vi "Initialize_Serial_Device_2.0.vi"(8 "error in (no error)":errorcluster, 10 "Enum":enum16{"Arduino Uno", "Pump", "Arduino Mega"}(ring), 11 "Data":T1 {"SystemVersion" items=["Standard", "XL"]; "Tap1" items=["Session Data", "Extended Setup", "Buffer", "Camera", "Dispenser", "Stats", "Connections"]; "I don't think is in use"."Light intensity" scale=0.0..100.0; "Camera settings"."Crop settings"."Cam2"."Rectangle 2"."Rotation" format="%.2f"; "Camera settings"."Crop settings"."Cam2"."Rectangle 2"."Left" scale=0.0..1024.0; "Camera settings"."Crop settings"."Cam2"."Rectangle 2"."Right" scale=0.0..1024.0; "Camera settings"."Crop settings"."Cam1"."Rectangle 1"."Rotation" format="%.2f"; "Camera settings"."Crop settings"."Cam1"."Rectangle 1"."Left" scale=0.0..1024.0; "Camera settings"."Crop settings"."Cam1"."Rectangle 1"."Right" scale=0.0..1024.0; "Camera settings"."Lens/camera settings"."Framerate" min=1; "Camera settings"."Lens/camera settings"."Max Framerate" min=1; "Camera settings"."Detection settings"."Sample size threshold" min=1; "Pump"."Flush Size" min=0 max=6000 step=100; "Ques"."Overload threshold" min=1; "Ques"."Image Save Queue Size" min=1; "Ques"."Image Process Queue Size" min=1}) -> (0 "error out":errorcluster, 2 "Connection":bool, 3 "Data 2":T1={"Camera 1"={"Camera1"="", "Cam 1"=FALSE, "CAM1 Model"=enum."a2A5328-15ucBAS", "Cam1 ID"=0}, "Camera 2"={"Camera2"="", "Cam 2"=FALSE, "CAM2 Model"=enum."a2A5328-15ucBAS", "Cam2 ID"=0}, "Image"={"Camera1_Img"=refnum, "Camera2_Img"=refnum, "Img1_Orig_Disp"=refnum, "Img2_Orig_Disp"=refnum, "Img1_Orig_RGB"=refnum, "Img2_Orig_RGB"=refnum, "Blue_Plane_Extract"=refnum, "Subtracted_Plane"=refnum, "Img1_Binary"=refnum, "Img2_Binary"=refnum, "Crop_Mask"=refnum, "Img1_Save"=refnum, "Img2_Save"=refnum, "Img1_Cali_Full"=refnum, "Img2_Cali_Full"=refnum, "Img1_Cali_Detect"=refnum, "Img2_Cali_Detect"=refnum}, "Ques"={"Cam 1 queue"=refnum, "Cam 2 queue"=refnum, "Cam 1 - save queue"=refnum, "Cam 2 - save queue"=refnum, "Image Process Queue Size"=500, "Image Save Queue Size"=500, "Overload threshold"=500, "Max large object threshold"=0}, "Arduino SRS"={"Pinch-valve"="", "Actuator"=FALSE, "Open(T)/Close(F)"=FALSE, "Arduino Uno"=""}, "Pump"={"Port"="", "Connection"=FALSE, "Flush Size"=0, "Command"="", "Pump Size"=enum."Large", "Pump"="", "Ready"=FALSE}, "Camera settings"={"Detection settings"={"Sample size threshold"=500, "Detection Region %"=30.0, "Timeout Sample"=200}, "Lens/camera settings"={"Aperture"=enum."Item 0", "Legacy Cam Attributes"=FALSE, "Max Framerate"=100, "Exposure Time"=1000.0, "Framerate"=15}, "Crop settings"={"Cam1"={"Rectangle 1"={"Left"=0, "Top"=0, "Right"=0, "Bottom"=0, "Rotation"=0.0}, "Camera Orientation 1"="", "Pixel to mm 1"=0.0}, "Cam2"={"Rectangle 2"={"Left"=0, "Top"=0, "Right"=0, "Bottom"=0, "Rotation"=0.0}, "Camera Orientation 2"="", "Pixel to mm 2"=0.0}}}, "Arduino ISS"={"Mega F3"="", "Phase3"=FALSE, "Barcode"="", "Sorting sys."=FALSE, "Initial size"=0.0, "Size Interval"=0.0, "Mun. of containers"=0.0, "Container nr."=0.0, "Arduino Mega"=""}, "Img_Capt"=FALSE, "Empty_Refill"=FALSE, "I don't think is in use"={"Light intensity"=100}, "Extended setup"={"Location"="Station", "Latitude"="Station", "Longitude"="Station", "Determiner"="Station", "Sex"="Station", "Station"="", "Collection date"=""}, "Main interface"={"Sample Name"="Test Sample", "Operator"="JFR", "Species Name"="", "Other Notes"=""}, "Tap1"=0, "SystemVersion"=0, "System Serial"="", "Exit"=FALSE, "Kuvette Full"=FALSE, "Core JKI"={"Current VI Reference"=refnum, "Close Panel on Exit?"=FALSE}, "Calibration"={"Calibration 1"=path "C:/Users/au540322/Desktop/IHS_Project/images/Debris/Debris_0/Debris_0_2019_06_01-23-32-49-686.PNG", "Calibration 2"=path "C:/Users/au540322/Desktop/IHS_Project/images/Debris/Debris_0/Debris_0_2019_06_01-23-32-49-686.PNG", "Detect 1"=path "C:/Users/au540322/Desktop/IHS_Project/images/Debris/Debris_0/Debris_0_2019_06_01-23-32-49-686.PNG", "Detect 2"=path "C:/Users/au540322/Desktop/IHS_Project/images/Debris/Debris_0/Debris_0_2019_06_01-23-32-49-686.PNG"}, "Auto Flush"=FALSE} {"SystemVersion" items=["Standard", "XL"]; "Tap1" items=["Session Data", "Extended Setup", "Buffer", "Camera", "Dispenser", "Stats", "Connections"]; "I don't think is in use"."Light intensity" scale=0.0..100.0; "Camera settings"."Crop settings"."Cam2"."Rectangle 2"."Rotation" format="%.2f"; "Camera settings"."Crop settings"."Cam2"."Rectangle 2"."Left" scale=0.0..1024.0; "Camera settings"."Crop settings"."Cam2"."Rectangle 2"."Right" scale=0.0..1024.0; "Camera settings"."Crop settings"."Cam1"."Rectangle 1"."Rotation" format="%.2f"; "Camera settings"."Crop settings"."Cam1"."Rectangle 1"."Left" scale=0.0..1024.0; "Camera settings"."Crop settings"."Cam1"."Rectangle 1"."Right" scale=0.0..1024.0; "Camera settings"."Lens/camera settings"."Framerate" min=1; "Camera settings"."Lens/camera settings"."Max Framerate" min=1; "Camera settings"."Detection settings"."Sample size threshold" min=1; "Pump"."Flush Size" min=0 max=6000 step=100; "Ques"."Overload threshold" min=1; "Ques"."Image Save Queue Size" min=1; "Ques"."Image Process Queue Size" min=1})   [LabVIEW 2024]
uses:
  controls/Data_JKI.ctl
  <vilib>/userDefined/High Color/IMAQdx.ctl
  <vilib>/vision/Image Controls.llb/IMAQ Image.ctl
  <vilib>/Instr/_visa.llb/VISA Find Search Mode.ctl
  b9f502e1-47a6-4cec-8472-59ce789a2094.vi
  24558789-6baa-4d89-876d-522026fff3d8.vi
  9ba94584-cf90-4084-937e-f244570da27e.vi
  19e22268-0b19-48d3-ab11-a72bc7dea378.vi
  <vilib>/regexp/Match Regular Expression.xnode
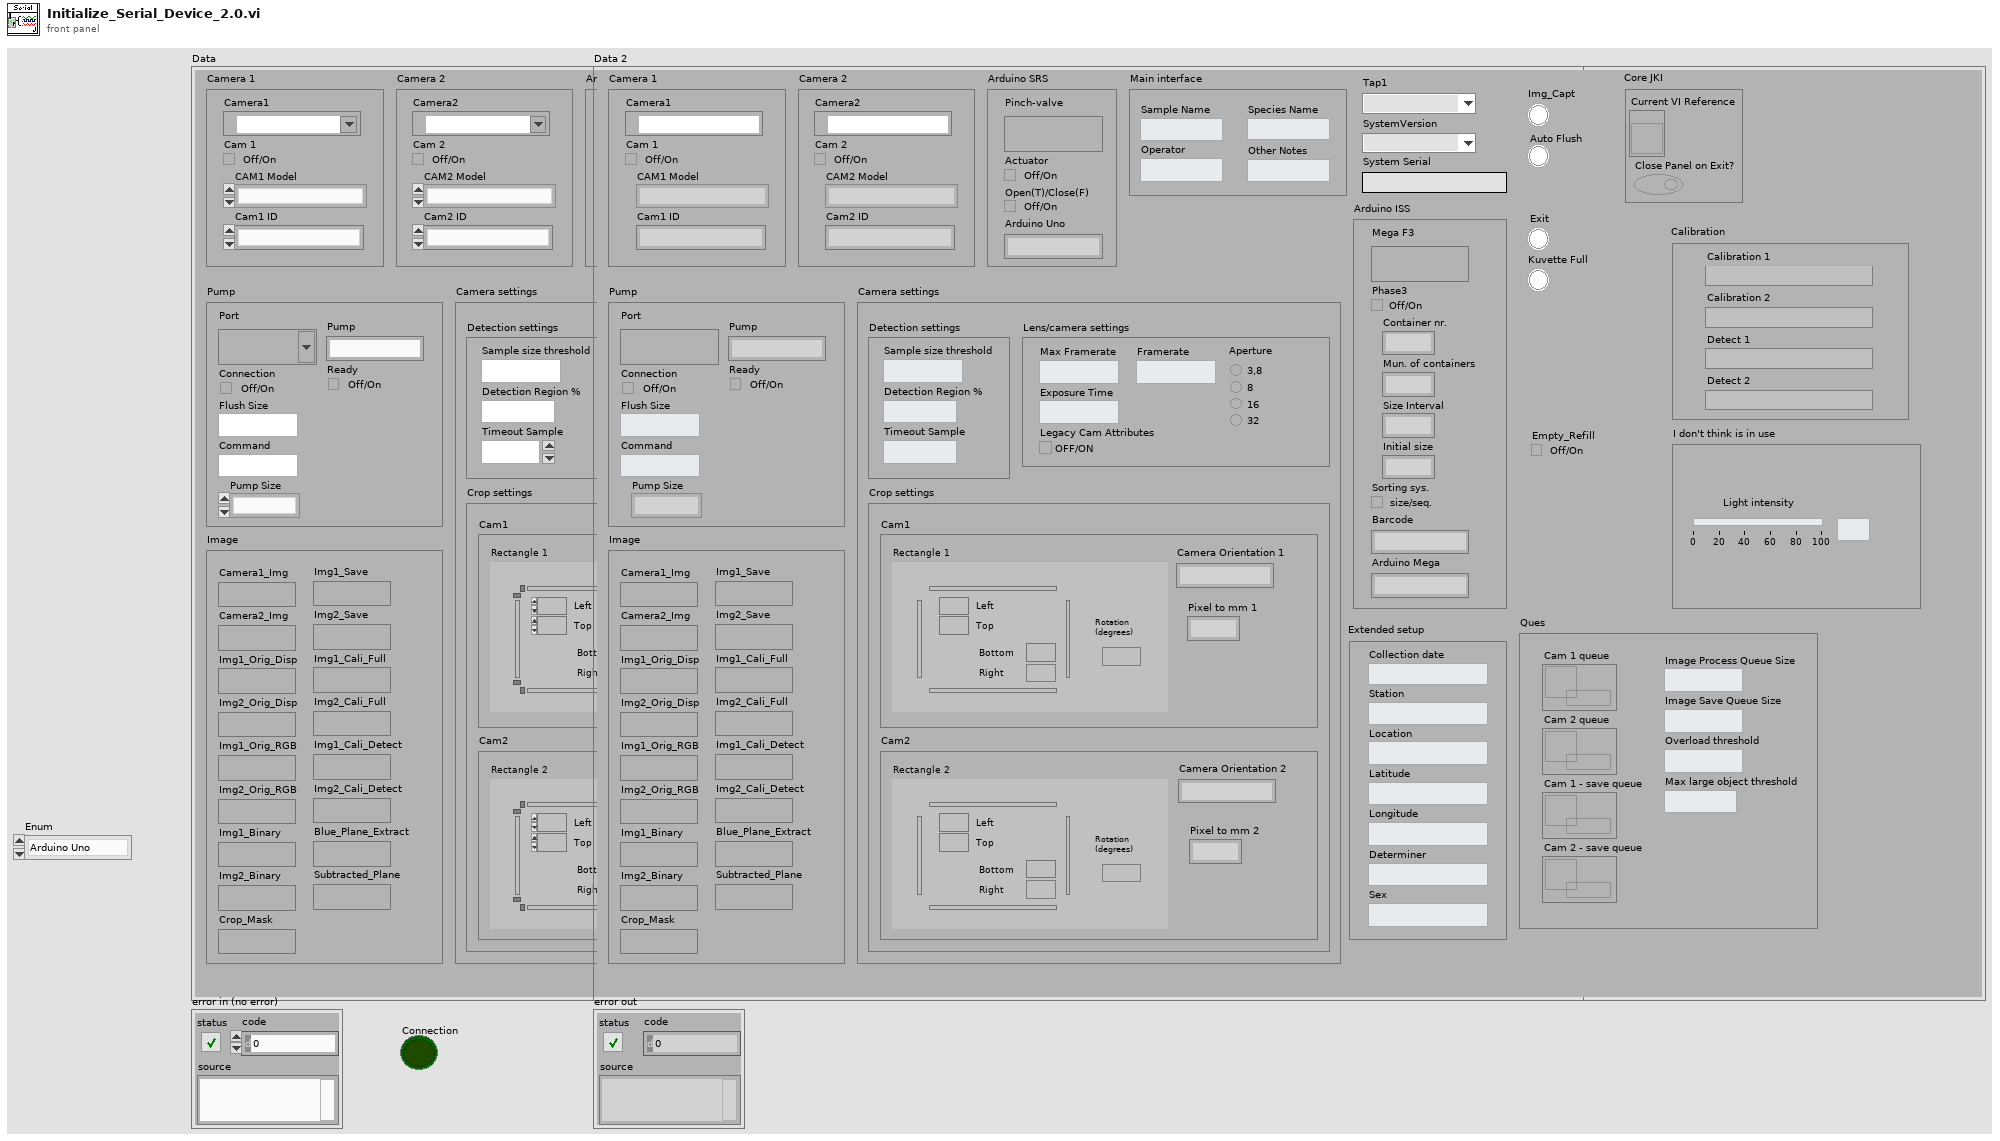
[diagram p1: front panel]
types:
  T1 = typedef "Data_JKI.ctl" = cluster{"Camera 1":cluster{"Camera1":T2, "Cam 1":bool, "CAM1 Model":enum16{"a2A5328-15ucBAS", "acA1920-155uc"}, "Cam1 ID":i32}, "Camera 2":cluster{"Camera2":T2, "Cam 2":bool, "CAM2 Model":enum16{"a2A5328-15ucBAS", "acA1920-155uc"}, "Cam2 ID":i32}, "Image":cluster{"Camera1_Img":T3, "Camera2_Img":T3, "Img1_Orig_Disp":T3, "Img2_Orig_Disp":T3, "Img1_Orig_RGB":T3, "Img2_Orig_RGB":T3, "Blue_Plane_Extract":T3, "Subtracted_Plane":T3, "Img1_Binary":T3, "Img2_Binary":T3, "Crop_Mask":T3, "Img1_Save":T3, "Img2_Save":T3, "Img1_Cali_Full":T3, "Img2_Cali_Full":T3, "Img1_Cali_Detect":T3, "Img2_Cali_Detect":T3}, "Ques":cluster{"Cam 1 queue":refnum<queue>, "Cam 2 queue":refnum<queue>, "Cam 1 - save queue":refnum<queue>, "Cam 2 - save queue":refnum<queue>, "Image Process Queue Size":i32, "Image Save Queue Size":i32, "Overload threshold":i32, "Max large object threshold":i32}, "Arduino SRS":cluster{"Pinch-valve":refnum<visa-resource-name>, "Actuator":bool, "Open(T)/Close(F)":bool, "Arduino Uno":string}, "Pump":cluster{"Port":refnum<visa-resource-name>, "Connection":bool, "Flush Size":i32, "Command":string, "Pump Size":enum16{"None", "Small", "Large"}, "Pump":string, "Ready":bool}, "Camera settings":cluster{"Detection settings":cluster{"Sample size threshold":i32, "Detection Region %":dbl, "Timeout Sample":i32}, "Lens/camera settings":cluster{"Aperture":enum32{"Item 0", "Item 1", "Item 2", "Item 3"}, "Legacy Cam Attributes":bool, "Max Framerate":i32, "Exposure Time":dbl, "Framerate":i32}, "Crop settings":cluster{"Cam1":cluster{"Rectangle 1":T4, "Camera Orientation 1":string, "Pixel to mm 1":dbl}, "Cam2":cluster{"Rectangle 2":T4, "Camera Orientation 2":string, "Pixel to mm 2":dbl}}}, "Arduino ISS":cluster{"Mega F3":refnum<visa-resource-name>, "Phase3":bool, "Barcode":string, "Sorting sys.":bool, "Initial size":dbl, "Size Interval":dbl, "Mun. of containers":dbl, "Container nr.":dbl, "Arduino Mega":string}, "Img_Capt":bool, "Empty_Refill":bool, "I don't think is in use":cluster{"Light intensity":i32}, "Extended setup":cluster{"Location":string, "Latitude":string, "Longitude":string, "Determiner":string, "Sex":string, "Station":string, "Collection date":string}, "Main interface":cluster{"Sample Name":string, "Operator":string, "Species Name":string, "Other Notes":string}, "Tap1":u16, "SystemVersion":u16, "System Serial":string, "Exit":bool, "Kuvette Full":bool, "Core JKI":cluster{"Current VI Reference":refnum<vi>, "Close Panel on Exit?":bool}, "Calibration":cluster{"Calibration 1":path, "Calibration 2":path, "Detect 1":path, "Detect 2":path}, "Auto Flush":bool}
  T2 = typedef "IMAQdx.ctl" = refnum<k21>
  T3 = typedef "IMAQ Image.ctl" = refnum<image>
  T4 = typedef "IMAQ Rectangle" = cluster{"Left":i32, "Top":i32, "Right":i32, "Bottom":i32, "Rotation":dbl}
  T5 = typedef "VISA Find Search Mode.ctl" = u32
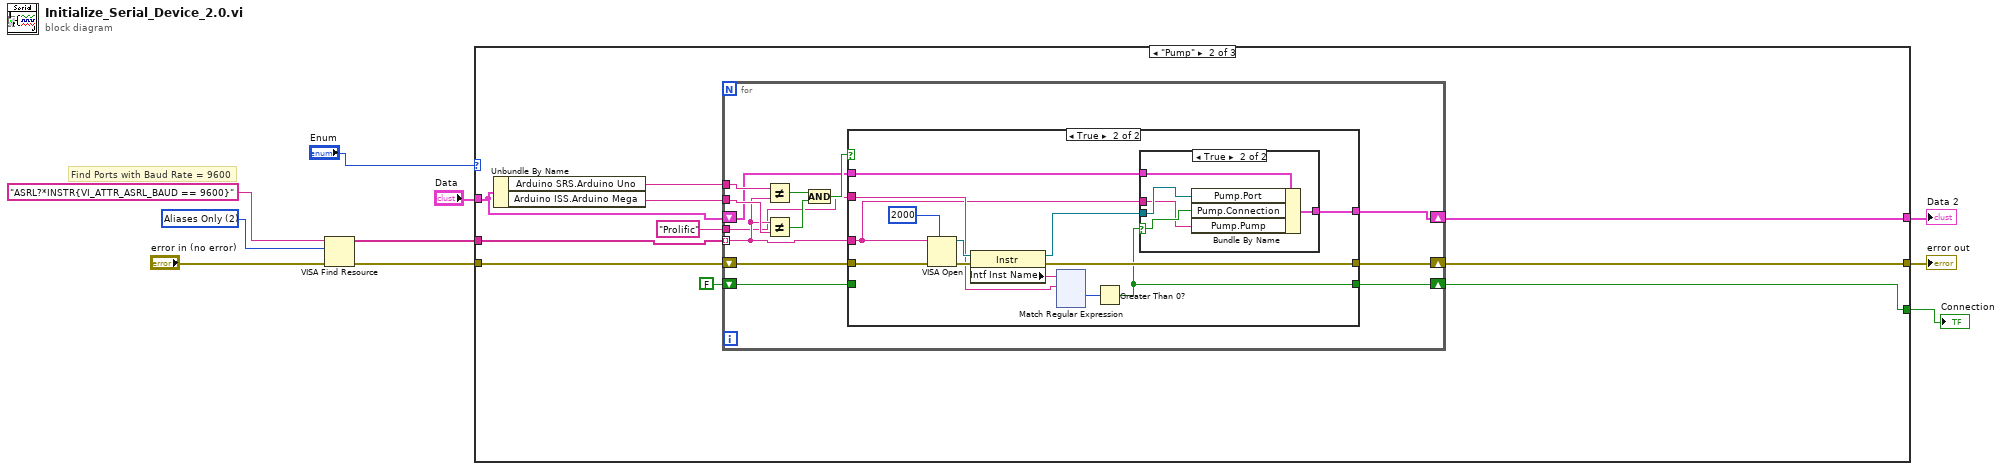
[diagram p0: block diagram]
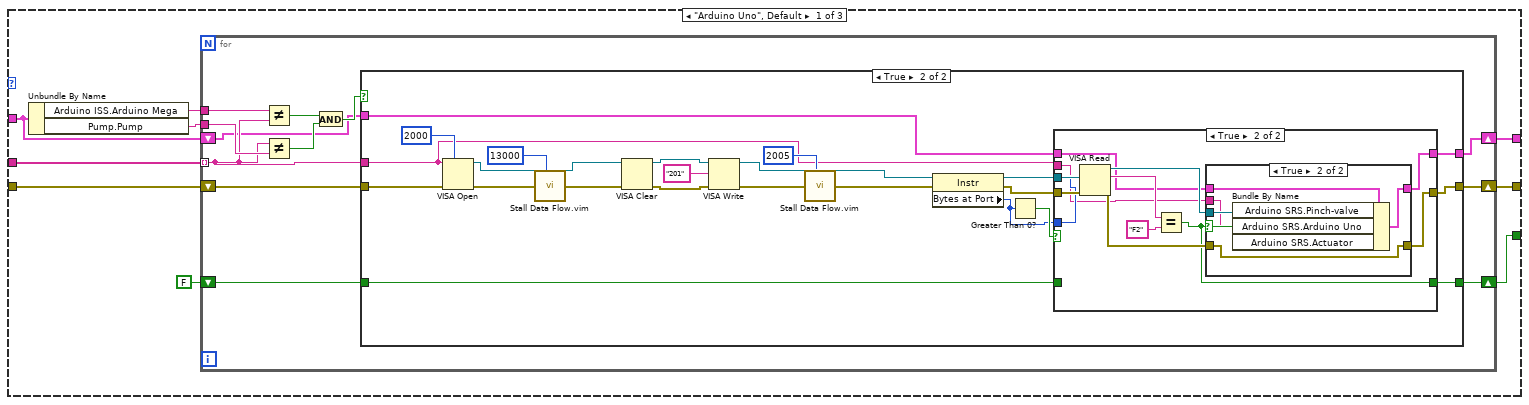
[diagram p2: hidden frame]
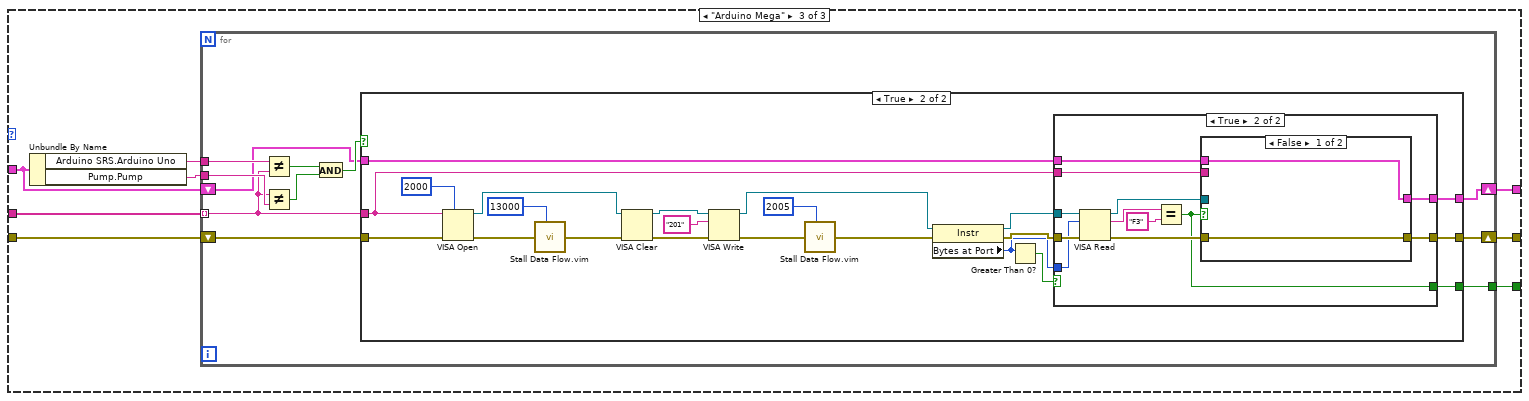
[diagram p8: hidden frame]
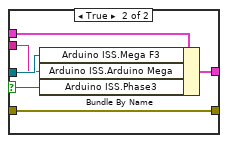
[diagram p11: hidden frame]
diagram:
  w10 = T5 2 items=["Canonical Names Only"=0, "Aliases Only"=2, "Include Matching Aliases"=3, "Include All Aliases"=4] ("Search Mode")
  # "Find Ports with Baud Rate = 9600"
  n1 = VISA Find Resource(8:"error in (no error)", 10:w10, 11:"ASRL?*INSTR{VI_ATTR_ASRL_BAUD == 9600}" ("expression (\"?*\")")) -> (0:w7:errorcluster, 3:w8:string[])  [unwired: 1 out]
  n2 = case shown="\"Pump\"" "Enum" {
    tunnel: w8 -> [w17 w90 w245]
    tunnel: w7 -> [w15 w86 w244]
    tunnel: "Data" -> [w16 w85 w246]
    tunnel: [w14 w84 w247] -> w5
    tunnel: [w13 w83 w248] -> w4
    tunnel: [w12 w82 w243] -> w1
    frame "Arduino Uno", Default {
      n3 = Unbundle By Name(w16) -> ("Arduino ISS.Arduino Mega"=w19:string, "Pump.Pump"=w18:string)
      n4 = for {
        tunnel: w17 -> [w29] mode=indexing
        tunnel: w19 -> [w31]
        tunnel: w18 -> [w30]
        shift-right: [w25] -> w14
        shift-left: w16 -> [w24]
        shift-right: [w22] -> w13
        shift-left: w15 -> [w23]
        shift-right: [w21] -> w12
        shift-left: FALSE -> [w20]
        n5 = Not Equal?(x=w31, y=w29) -> (x != y?=w28:bool)
        n6 = Not Equal?(x=w29, y=w30) -> (x != y?=w27:bool)
        n7 = And(x=w28, y=w27) -> (x .and. y?=w26:bool)
        n8 = case shown="True" w26 {
          tunnel: w29 -> [_ w38]
          tunnel: w24 -> [w34 w39]
          tunnel: [w34 w37] -> w25
          tunnel: w23 -> [w33 w43]
          tunnel: [w33 w40] -> w22
          tunnel: [w32 w36] -> w21
          tunnel: w20 -> [w32 w35]
          frame False {
          }
          frame True {
            n9 = VISA Open(timeout (0)=u32 2000 ("VISA Open timeout (0)"), error in (no error)=w43, VISA resource name=w38) -> (VISA resource name=w42:refnum<visa-resource-name>, error out=w41:errorcluster)  [unwired: 2 in]
            n10 = call "Stall Data Flow.vim"("value in"=w41, "milliseconds to wait"=u32 13000) -> ("value out"=w46:errorcluster)  [unwired: 1 out]
            n11 = VISA Clear(VISA resource name=w42, error in (no error)=w46) -> (VISA resource name out=w56:refnum<visa-resource-name>, error out=w57:errorcluster)
            n12 = VISA Write(VISA resource name=w56, write buffer="201", error in (no error)=w57) -> (VISA resource name out=w54:refnum<visa-resource-name>, error out=w49:errorcluster)  [unwired: 1 out]
            n13 = call "Stall Data Flow.vim"("value in"=w49, "milliseconds to wait"=u32 2005) -> ("value out"=w48:errorcluster)  [unwired: 1 out]
            n14 = property class="Instr"(reference=w54, error in=w48) -> (reference out=w52:refnum<visa-resource-name>, error out=w51:errorcluster, "Bytes at Port"=w50:u32)
            n15 = Greater Than 0?(x=w50) -> (x > 0?=w53:bool)
            n16 = case shown="True" w53 {
              tunnel: w52 -> [_ w72]
              tunnel: w51 -> [w59 w71]
              tunnel: w50 -> [_ w70]
              tunnel: [w59 w66] -> w40
              tunnel: w39 -> [w60 w64]
              tunnel: w38 -> [_ w63]
              tunnel: [w60 w62] -> w37
              tunnel: [w58 w61] -> w36
              tunnel: w35 -> [w58 _]
              frame False {
              }
              frame True {
                n17 = VISA Read(VISA resource name=w72, byte count=w70, error in (no error)=w71) -> (VISA resource name out=w65:refnum<visa-resource-name>, read buffer=w69:string, error out=w67:errorcluster)  [unwired: 1 out]
                n18 = Equal?(x=w69, y="F2") -> (x = y?=w61:bool)
                n19 = case shown="True" w61 {
                  selector: w61 -> [_ w77]
                  tunnel: [w73 w80] -> w66
                  tunnel: w67 -> [w73 w80]
                  tunnel: w65 -> [_ w78]
                  tunnel: w64 -> [w74 w79]
                  tunnel: w63 -> [_ w76]
                  tunnel: [w74 w75] -> w62
                  frame False {
                  }
                  frame True {
                    n20 = Bundle By Name(cluster=w79, "Arduino SRS.Pinch-valve"=w78, "Arduino SRS.Arduino Uno"=w76, "Arduino SRS.Actuator"=w77) -> (w75:T1)
                  }
                }
              }
            }
          }
        }
      }
    }
    frame "Pump" {
      n21 = Unbundle By Name(w85) -> ("Arduino SRS.Arduino Uno"=w89:string, "Arduino ISS.Arduino Mega"=w87:string)
      n22 = for {
        tunnel: w90 -> [w101] mode=indexing
        tunnel: w89 -> [w103]
        tunnel: "Prolific" -> [w97]
        tunnel: w87 -> [w102]
        shift-right: [w96] -> w84
        shift-left: w85 -> [w95]
        shift-right: [w93] -> w83
        shift-left: w86 -> [w94]
        shift-right: [w92] -> w82
        shift-left: FALSE -> [w91]
        n23 = Not Equal?(x=w103, y=w101) -> (x != y?=w100:bool)
        n24 = Not Equal?(x=w101, y=w102) -> (x != y?=w99:bool)
        n25 = And(x=w100, y=w99) -> (x .and. y?=w98:bool)
        n26 = case shown="True" w98 {
          tunnel: w101 -> [_ w108]
          tunnel: w97 -> [_ w114]
          tunnel: w95 -> [w106 w113]
          tunnel: [w106 w111] -> w96
          tunnel: w94 -> [w105 w110]
          tunnel: [w105 w109] -> w93
          tunnel: [w104 w107] -> w92
          tunnel: w91 -> [w104 _]
          frame False {
          }
          frame True {
            n27 = VISA Open(timeout (0)=u32 2000 ("VISA Open timeout (0)"), error in (no error)=w110, VISA resource name=w108) -> (VISA resource name=w119:refnum<visa-resource-name>, error out=w116:errorcluster)  [unwired: 2 in]
            n28 = property class="Instr"(reference=w119, error in=w116) -> (reference out=w112:refnum<visa-resource-name>, error out=w109:errorcluster, "Intf Inst Name"=w115:string)
            n29 = xnode "Match Regular Expression"("input string"=w115, "regular expression"=w114) -> ("offset past match"=w118:i32)  [unwired: 4 in, 4 out]
            n30 = Greater Than 0?(x=w118) -> (x > 0?=w107:bool)
            n31 = case shown="True" w107 {
              selector: w107 -> [_ w124]
              tunnel: w113 -> [w120 w125]
              tunnel: w112 -> [_ w123]
              tunnel: [w120 w122] -> w111
              tunnel: w108 -> [_ w121]
              frame False {
              }
              frame True {
                n32 = Bundle By Name(cluster=w125, "Pump.Port"=w123, "Pump.Connection"=w124, "Pump.Pump"=w121) -> (w122:T1)
              }
            }
          }
        }
      }
    }
    frame "Arduino Mega" {
      n33 = Unbundle By Name(w246) -> ("Arduino SRS.Arduino Uno"=w250:string, "Pump.Pump"=w249:string)
      n34 = for {
        tunnel: w245 -> [w259] mode=indexing
        tunnel: w250 -> [w261]
        tunnel: w249 -> [w260]
        shift-right: [w255] -> w247
        shift-left: w246 -> [w254]
        shift-right: [w252] -> w248
        shift-left: w244 -> [w253]
        tunnel: [w251] -> w243
        n35 = Not Equal?(x=w261, y=w259) -> (x != y?=w258:bool)
        n36 = Not Equal?(x=w259, y=w260) -> (x != y?=w257:bool)
        n37 = And(x=w258, y=w257) -> (x .and. y?=w256:bool)
        n38 = case shown="True" w256 {
          selector: w256 -> [w262 _]
          tunnel: w259 -> [_ w267]
          tunnel: w254 -> [w264 w268]
          tunnel: [w264 w266] -> w255
          tunnel: w253 -> [w263 w272]
          tunnel: [w263 w269] -> w252
          tunnel: [w262 w265] -> w251
          frame False {
          }
          frame True {
            n39 = VISA Open(timeout (0)=u32 2000 ("VISA Open timeout (0)"), error in (no error)=w272, VISA resource name=w267) -> (VISA resource name=w271:refnum<visa-resource-name>, error out=w270:errorcluster)  [unwired: 2 in]
            n40 = call "Stall Data Flow.vim"("value in"=w270, "milliseconds to wait"=u32 13000) -> ("value out"=w275:errorcluster)  [unwired: 1 out]
            n41 = VISA Clear(VISA resource name=w271, error in (no error)=w275) -> (VISA resource name out=w285:refnum<visa-resource-name>, error out=w286:errorcluster)
            n42 = VISA Write(VISA resource name=w285, write buffer="201", error in (no error)=w286) -> (VISA resource name out=w283:refnum<visa-resource-name>, error out=w278:errorcluster)  [unwired: 1 out]
            n43 = call "Stall Data Flow.vim"("value in"=w278, "milliseconds to wait"=u32 2005) -> ("value out"=w277:errorcluster)  [unwired: 1 out]
            n44 = property class="Instr"(reference=w283, error in=w277) -> (reference out=w281:refnum<visa-resource-name>, error out=w280:errorcluster, "Bytes at Port"=w279:u32)
            n45 = Greater Than 0?(x=w279) -> (x > 0?=w282:bool)
            n46 = case shown="True" w282 {
              selector: w282 -> [w287 _]
              tunnel: w281 -> [_ w301]
              tunnel: w280 -> [w288 w300]
              tunnel: w279 -> [_ w299]
              tunnel: [w288 w295] -> w269
              tunnel: w268 -> [w289 w293]
              tunnel: w267 -> [_ w292]
              tunnel: [w289 w291] -> w266
              tunnel: [w287 w290] -> w265
              frame False {
              }
              frame True {
                n47 = VISA Read(VISA resource name=w301, byte count=w299, error in (no error)=w300) -> (VISA resource name out=w294:refnum<visa-resource-name>, read buffer=w298:string, error out=w296:errorcluster)  [unwired: 1 out]
                n48 = Equal?(x=w298, y="F3") -> (x = y?=w290:bool)
                n49 = case shown="False" w290 {
                  selector: w290 -> [_ w304]
                  tunnel: [w302 w309] -> w295
                  tunnel: w296 -> [w302 w309]
                  tunnel: w294 -> [_ w307]
                  tunnel: w293 -> [w303 w308]
                  tunnel: w292 -> [_ w306]
                  tunnel: [w303 w305] -> w291
                  frame False {
                  }
                  frame True {
                    n50 = Bundle By Name(cluster=w308, "Arduino ISS.Mega F3"=w307, "Arduino ISS.Arduino Mega"=w306, "Arduino ISS.Phase3"=w304) -> (w305:T1)
                  }
                }
              }
            }
          }
        }
      }
    }
  }
  "Data 2" <- w5
  "error out" <- w4
  "Connection" <- w1
